vi "miclose.vi"(1 "错误输入（无错误）":errorcluster, 2 "VISA资源名称":refnum<visa-resource-name>) -> (0 "错误输出":errorcluster)   [LabVIEW 2017]
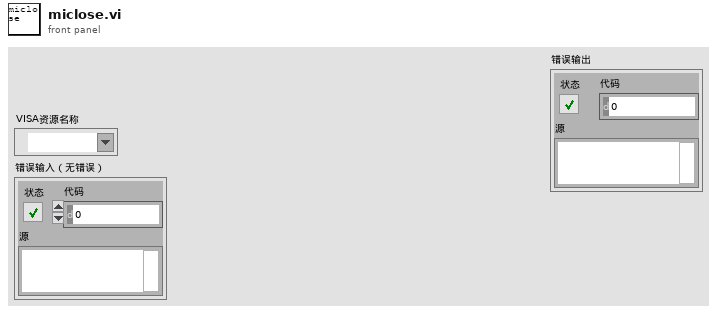
[diagram p1: front panel]
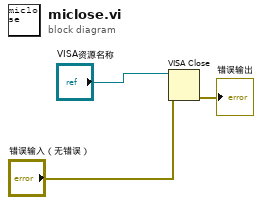
[diagram p0: block diagram]
diagram:
  n1 = VISA Close(VISA resource name="VISA资源名称", error in (no error)="错误输入（无错误）") -> (error out=→"错误输出":errorcluster)
